vi "InitializeOpenCVIP.vi"(1 "dataDirectory":string, 2 "Image processing preferences":T1={"scale"=0.5, "elSizeImOpen"=21, "thresholdBinarizationBody"=0.65, "thresholdBinarizationWings"=0.2, "minWingArea"=20000, "quantile"=0.05, "elSizeImOpenIdent1"=15, "elSizeImOpenIdent2"=21, "thresholdBinarizationIdent"=0.65, "elSizeImHMin"=6, "raiseParImHMin"=0.33, "focus limit"=50, "maxAllowedRotation"=30.0, "elSizeImClose"=3, "numIterImClose"=3, "symmetryMinOverlapBody"=95.0, "symmetryMinOverlapWings"=85.0, "thresholdReflectionCheck"=0.99, "elSizeReflection"=7, "maxReflectionArea"=2000, "upSideDownCheck"=0.99}) -> (0 "return type":i32)   [LabVIEW 2012]
uses:
  OpenCvGlobals.vi
  <userlib>/OpenCVImProc/CatWalkLabviewDLLd.dll
  <userlib>/OpenCVImProc/CatWalkLabviewDLL.dll
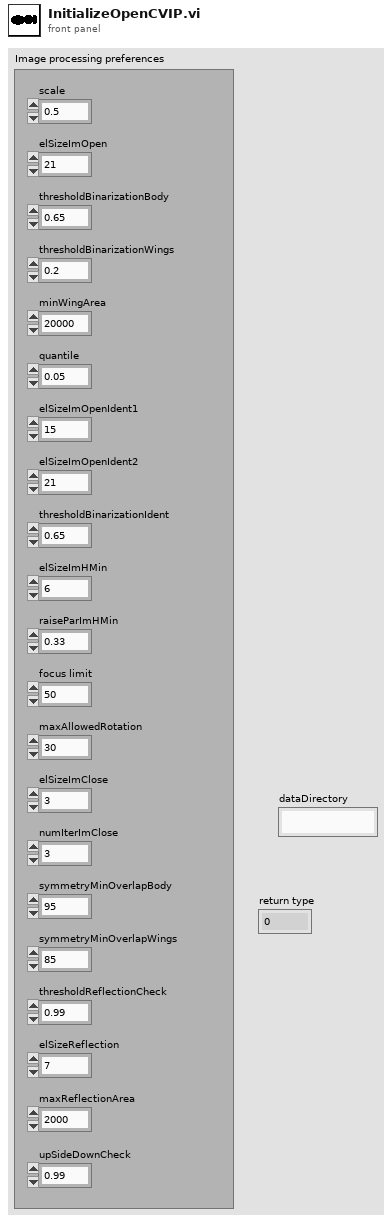
[diagram p1: front panel]
types:
  T1 = cluster{"scale":sgl, "elSizeImOpen":i32, "thresholdBinarizationBody":sgl, "thresholdBinarizationWings":sgl, "minWingArea":i32, "quantile":sgl, "elSizeImOpenIdent1":i32, "elSizeImOpenIdent2":i32, "thresholdBinarizationIdent":sgl, "elSizeImHMin":i32, "raiseParImHMin":sgl, "focus limit":i32, "maxAllowedRotation":sgl, "elSizeImClose":i32, "numIterImClose":i32, "symmetryMinOverlapBody":sgl, "symmetryMinOverlapWings":sgl, "thresholdReflectionCheck":sgl, "elSizeReflection":i32, "maxReflectionArea":i32, "upSideDownCheck":sgl}
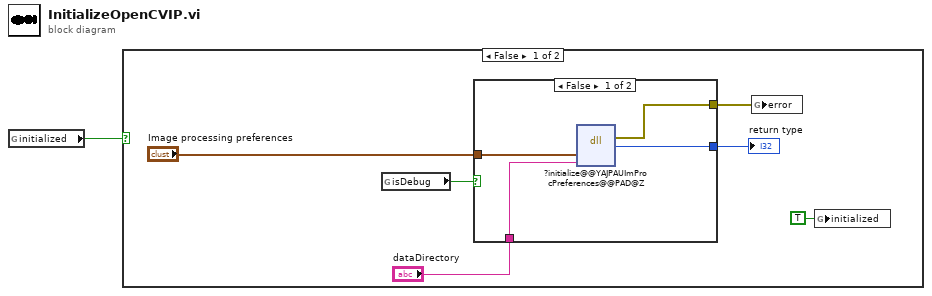
[diagram p0: block diagram]
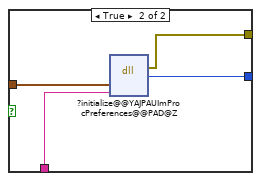
[diagram p2: hidden frame]
diagram:
  n1 = global read "OpenCvGlobals.vi" "initialized"() -> (w1:bool)
  n2 = case shown="False" w1 {
    frame False {
      n3 = global read "OpenCvGlobals.vi" "isDebug"() -> (w4:bool)
      n4 = case shown="False" w4 {
        tunnel: "Image processing preferences" -> [w10 w15]
        tunnel: [w11 w14] -> w5
        tunnel: [w9 w13] -> w6
        tunnel: "dataDirectory" -> [w8 w12]
        frame False {
          n5 = dll-call lib="C:/Program Files (x86)/National Instruments/LabVIEW 2012/user.lib/OpenCVImProc/CatWalkLabviewDLL.dll" fn="?initialize@@YAJPAUImProcPreferences@@PAD@Z"("prefIn"=w10, "dataDirectory"=w8) -> (error out=w9:errorcluster, "return type"=w11:i32)  [unwired: 5 in, 1 out]
        }
        frame True {
          n6 = dll-call lib="C:/Program Files (x86)/National Instruments/LabVIEW 2012/user.lib/OpenCVImProc/CatWalkLabviewDLLd.dll" fn="?initialize@@YAJPAUImProcPreferences@@PAD@Z"("prefIn"=w15, "dataDirectory"=w12) -> (error out=w13:errorcluster, "return type"=w14:i32)  [unwired: 5 in, 1 out]
        }
      }
      "return type" <- w5
      n7 = global write "OpenCvGlobals.vi" "error"(w6) -> ()
      n8 = global write "OpenCvGlobals.vi" "initialized"(TRUE ("initialized")) -> ()
    }
    frame True {
    }
  }
